vi "checkin.vi"(8 "error in (no error)":errorcluster, 11 "GenericDAQ in":refnum<class "GenericDAQ.lvclass">) -> (0 "error out":errorcluster, 3 "GenericDAQ out":refnum<class "GenericDAQ.lvclass">)   [LabVIEW 2010, in "GenericDAQ.lvclass"]
uses:
  GenericDAQ.lvclass
  common/classes/GenericToplevelComponent/GenericToplevelComponent/GenericToplevelComponent.lvclass
  class_data.vi
  common/classes/GenericComponent/GenericComponent/GenericComponent.lvclass
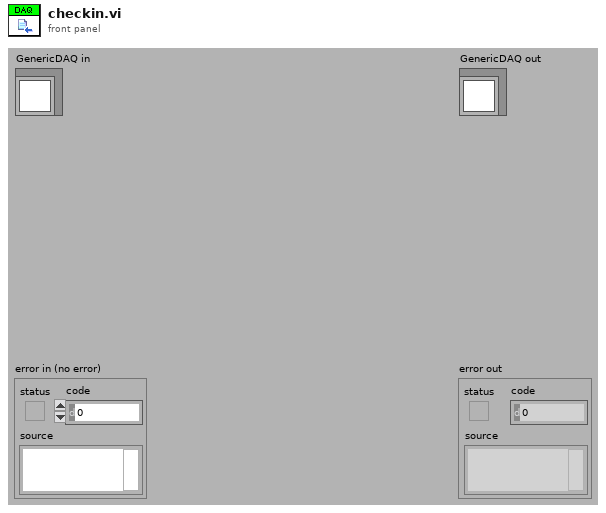
[diagram p1: front panel]
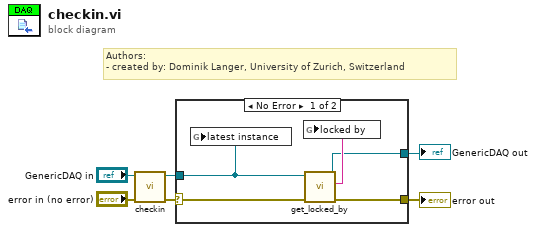
[diagram p0: block diagram]
diagram:
  # "Authors: \n- created by: Dominik Langer, University of Zurich, Switzerland"
  n1 = call-parent "checkin.vi"("error in (no error)"="error in (no error)", "GenericPlugin in"="GenericDAQ in") -> ("error out"=w1:errorcluster, "GenericPlugin out"=w3:refnum<class "GenericDAQ.lvclass">)  [unwired: 8 in]
  n2 = case shown="No Error" w1 {
    selector: w1 -> [w9 w13]
    tunnel: [w7 w13] -> w5
    tunnel: [w10 w12] -> w6
    tunnel: w3 -> [w8 w12]
    frame No Error {
      n3 = global write "class_data.vi" "latest instance"(w8) -> ()
      n4 = call "get_locked_by.vi"("error in (no error)"=w9, "GenericPlugin.lvclass in"=w8) -> ("error out"=w7:errorcluster, "locked by"=w11:string, "GenericPlugin.lvclass out"=w10:refnum<class "GenericDAQ.lvclass">)  [unwired: 7 out]
      n5 = global write "class_data.vi" "locked by"(w11) -> ()
    }
    frame Error {
    }
  }
  "error out" <- w5
  "GenericDAQ out" <- w6
